vi "Front Panel Tyler.vi"() -> ()   [LabVIEW 2017, in "LD Reading.lvclass"]
uses:
  LD Reading.lvclass
  Reference Channel Intensities.ctl
  Sample Channel Intensities.ctl
  Realtime Output.ctl
  Average Data.ctl
  LD Reading.lvclass/LD Reading.ctl
  <vilib>/Utility/file.llb/Write Delimited Spreadsheet (string).vi
panel:
  out "Sample Averages":T1
  out "Reference Averages":T1
  in  "Export Data":bool
  out "Data Collection Progress":u8(slide) scale=0.0..100.0
  out "Current Phase":string
  in  "Data graphs":enum32{"Data", "Miscellaneous Data"}(tab)
  out "Diode/PMT":cluster{dbl[], dbl[]}(graph)
  out "RMS Voltage (mV)":cluster{dbl[], dbl[]}(graph)
  out "Photodiode Voltage  (V)":cluster{dbl[], dbl[]}(graph)
  out "PMT Voltage (V)":cluster{dbl[], dbl[]}(graph)
  in  "Data Collection Mode":enum32{"Reference", "Sample"}(radio)
  in  "Selected Sample Channel":enum32{"Channel 1", "Channel 2", "Channel 3"}(radio)
  in  "Selected Reference Channel":enum32{"Channel 1", "Channel 2", "Channel 3"}(radio)
  out "Realtime Output":T2
  out "Sample Analysis":T3
  out "Reference Analysis":T4
  in  "Correction Factor":dbl
  out "Finished":bool
  in  "Output Filename (stem)":path
  in  "Stop Data Collection":bool
  in  "Save Measurements?":bool
  out "Running":bool
  in  "Number of Data Points":dbl
  in  "Data Interval (s)":dbl
  in  "Collect Data":bool
  in  "stop":bool
  # "Data Collection Parameters"
  # "Experiment Control"
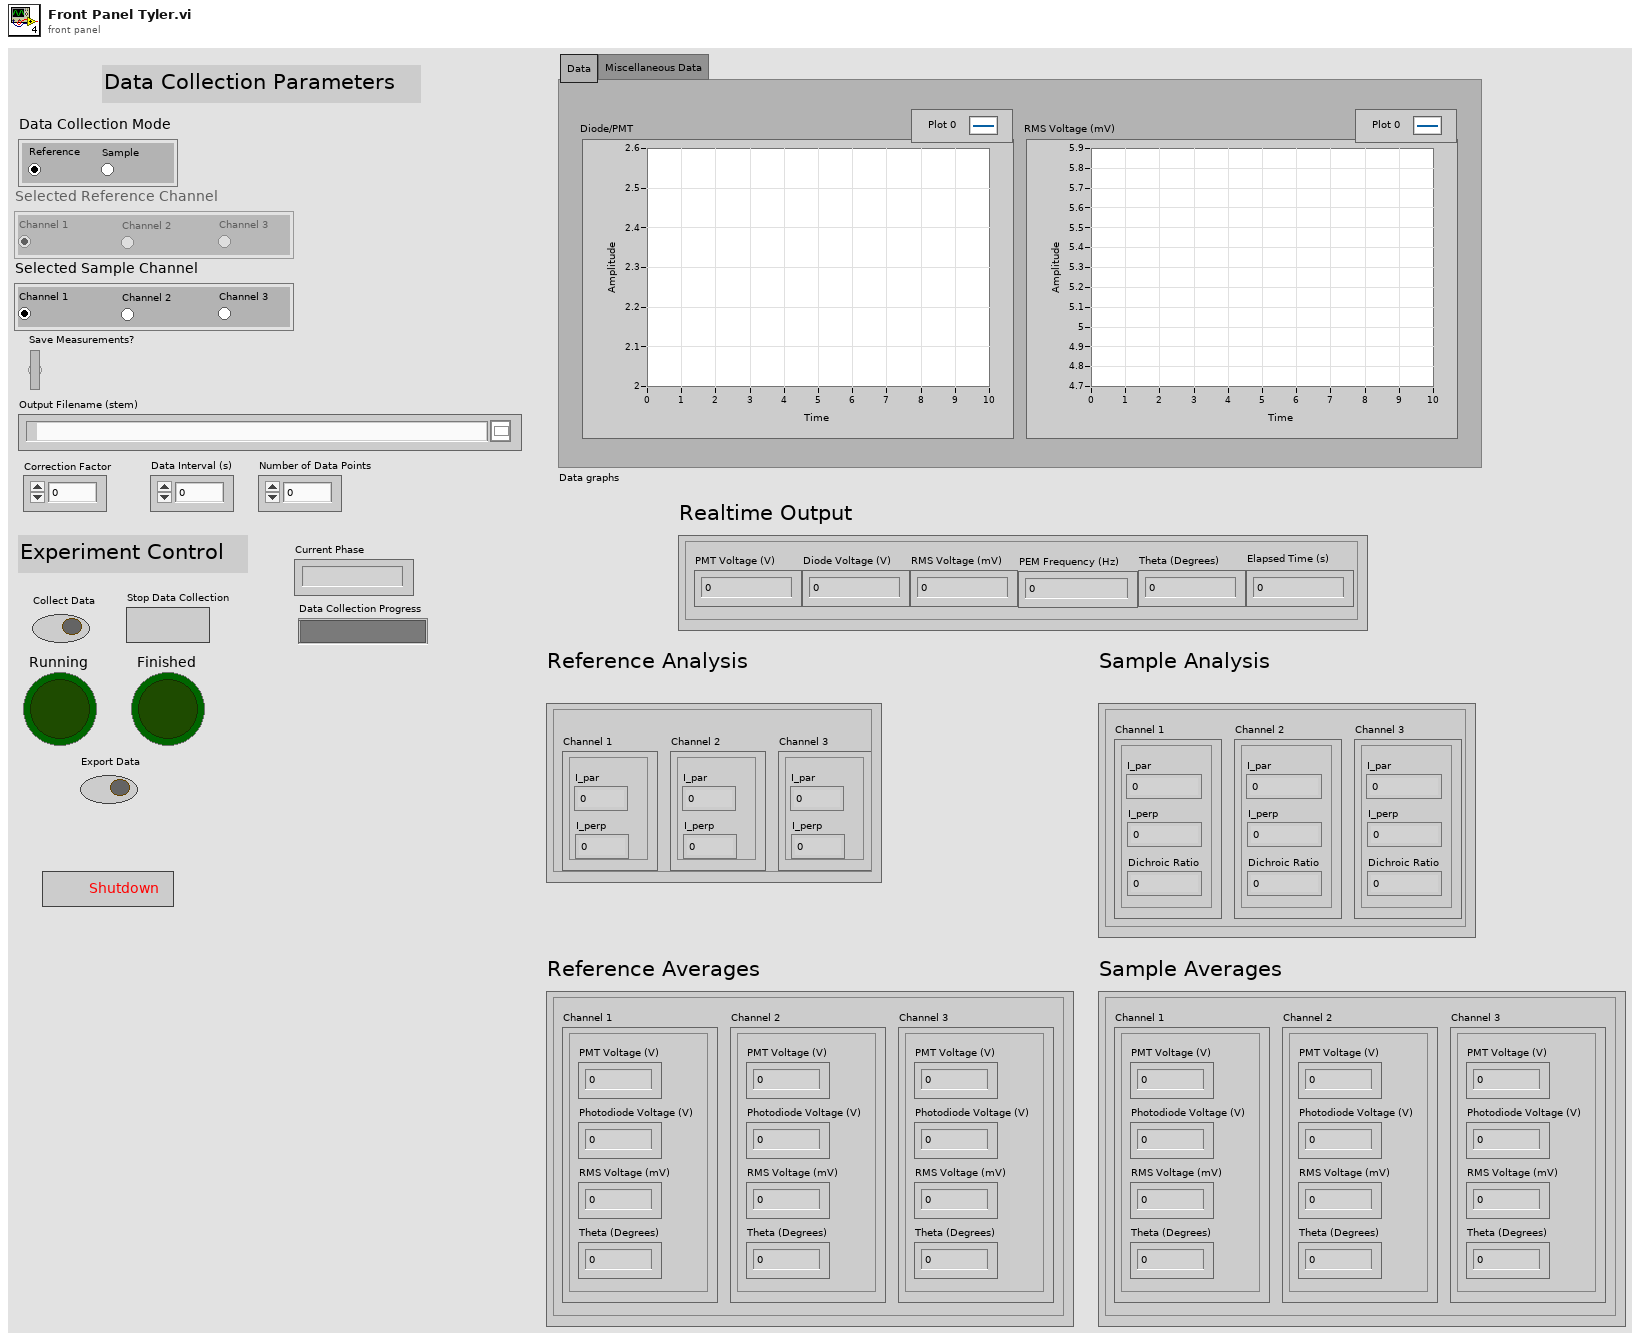
[diagram p1: front panel]
types:
  T1 = typedef "Average Data.ctl" = cluster{"Channel 1":cluster{"PMT Voltage (V)":dbl, "Photodiode Voltage (V)":dbl, "RMS Voltage (mV)":dbl, "Theta (Degrees)":dbl}, "Channel 2":cluster{"PMT Voltage (V)":dbl, "Photodiode Voltage (V)":dbl, "RMS Voltage (mV)":dbl, "Theta (Degrees)":dbl}, "Channel 3":cluster{"PMT Voltage (V)":dbl, "Photodiode Voltage (V)":dbl, "RMS Voltage (mV)":dbl, "Theta (Degrees)":dbl}}
  T2 = typedef "Realtime Output.ctl" = cluster{"Elapsed Time (s)":dbl, "PMT Voltage (V)":dbl, "Diode Voltage (V)":dbl, "RMS Voltage (mV)":dbl, "Theta (Degrees)":dbl, "PEM Frequency (Hz)":dbl}
  T3 = typedef "Sample Channel Intensities.ctl" = cluster{"Channel 1":cluster{"I_par":dbl, "I_perp":dbl, "Dichroic Ratio":dbl}, "Channel 2":cluster{"I_par":dbl, "I_perp":dbl, "Dichroic Ratio":dbl}, "Channel 3":cluster{"I_par":dbl, "I_perp":dbl, "Dichroic Ratio":dbl}}
  T4 = typedef "Reference Channel Intensities.ctl" = cluster{"Channel 1":cluster{"I_par":dbl, "I_perp":dbl}, "Channel 2":cluster{"I_par":dbl, "I_perp":dbl}, "Channel 3":cluster{"I_par":dbl, "I_perp":dbl}}
  T5 = enum8{"Enabled", "Disabled", "Disabled and Grayed Out"}
  T6 = cluster{dbl[], dbl[], dbl[], dbl[], dbl[], dbl[], dbl[]}
  T7 = cluster{"RMS Voltage Array":dbl[], "Photodiode Voltage Array":dbl[], "PMT Voltage Array":dbl[], "Diode/PMT Ratio Array":dbl[], "Time Array":dbl[], "PEM Frequency Array":dbl[], "Theta Array":dbl[]}
  T8 = cluster{"PMT Voltage (V)":dbl, "Photodiode Voltage (V)":dbl, "RMS Voltage (mV)":dbl, "Theta (Degrees)":dbl}
  T9 = cluster{"I_par":dbl, "I_perp":dbl, "Dichroic Ratio":dbl}
  T10 = typedef "NI_Matrix.lvlib/RealMatrix.ctl" = dbl[][]
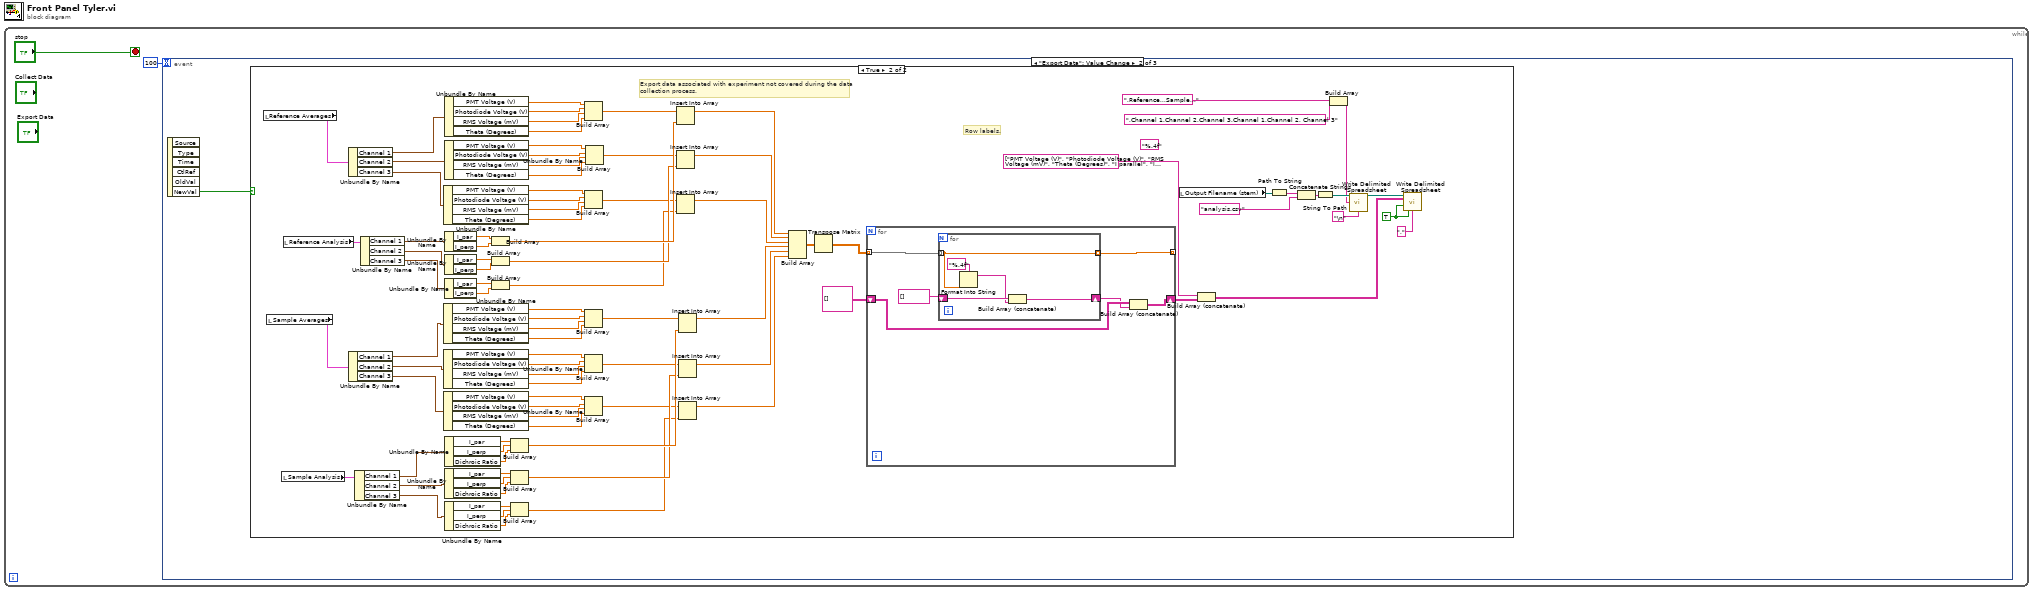
[diagram p0: block diagram]
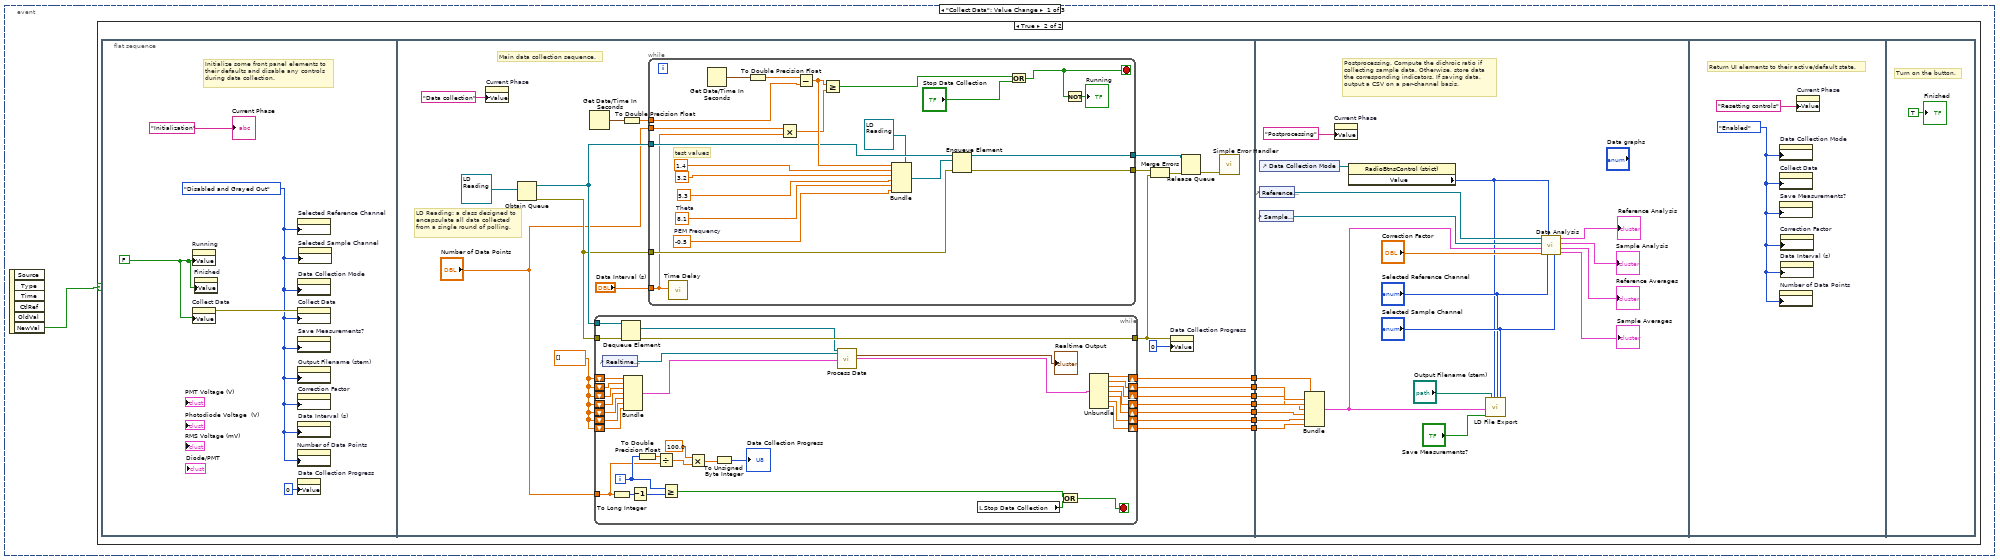
[diagram p2: hidden frame]
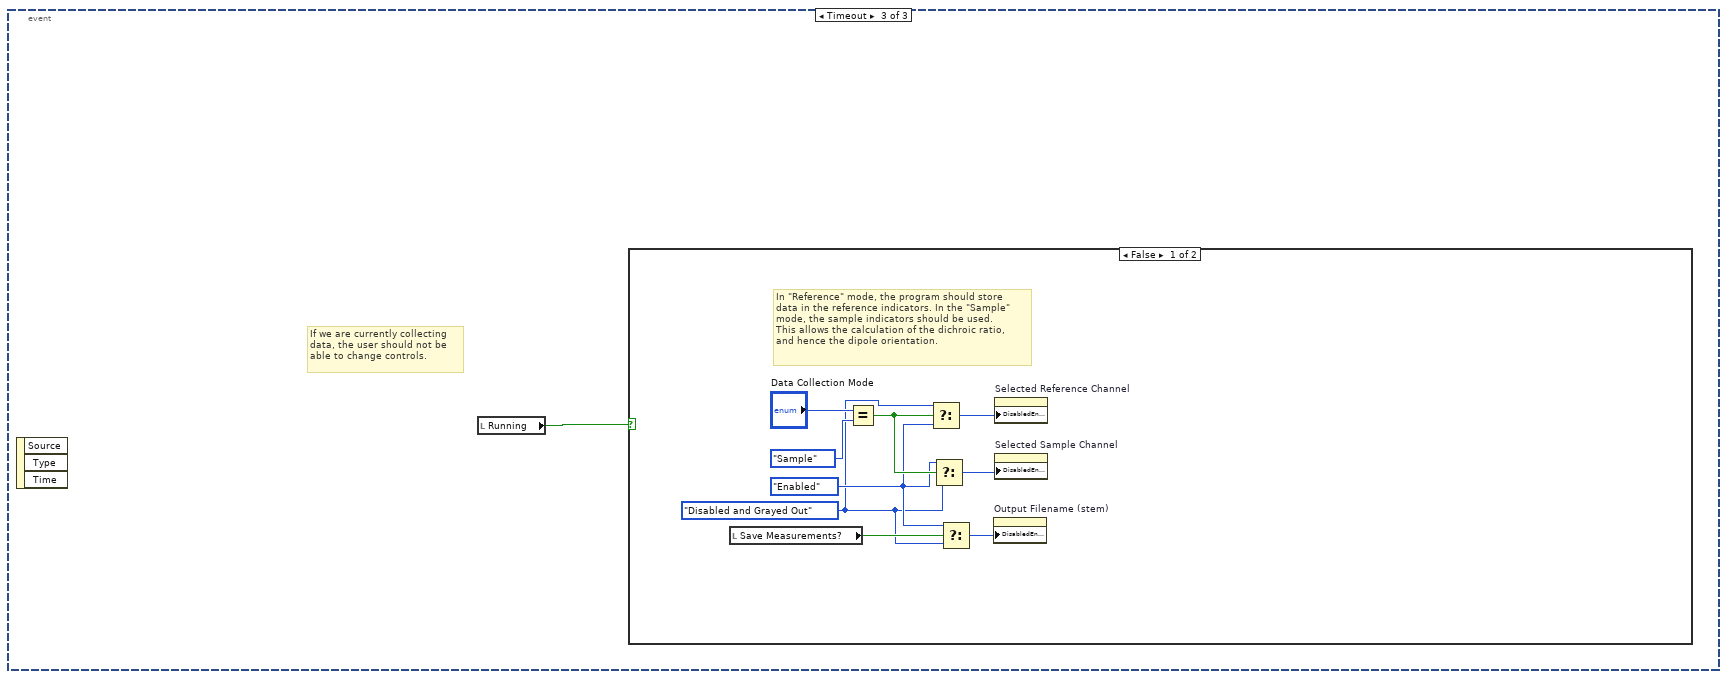
[diagram p5: hidden frame]
diagram:
  n1 = while {
    stop <- "stop" stop-if-true
    n2 = event shown="[1] \"Export Data\": Value Change" {
      selector: _ -> [_ _ _]
      dyn-events: _ -> [_ _ _]
      timeout: 100 -> [_ _ _]
      event "Collect Data": Value Change {
        n3 = event-data() -> ("NewVal"=w3:bool)  [unwired: 1 in, 5 out]
        n4 = case shown="True" w3 {
          frame False {
          }
          frame True {
            n5 = flat-sequence {
              tunnel: [w25] -> w10
              tunnel: [w24] -> w9
              tunnel: [w23] -> w8
              tunnel: [w26] -> w7
              tunnel: [w22] -> w6
              tunnel: [w21] -> w5
              tunnel: [w16] -> w4
              tunnel: w10 -> [w111]
              tunnel: w9 -> [w110]
              tunnel: w8 -> [w109]
              tunnel: w7 -> [w112]
              tunnel: w6 -> [w108]
              tunnel: w5 -> [w107]
              tunnel: w4 -> [w106]
              frame #0 {
                w13 = T5."Disabled and Grayed Out" ("Disabled")
                w15 = FALSE
                # "Initialize some front panel elements to \ntheir defaults and disable any controls \nduring data collection."
                n6 = property on="Running" class="Bool (strict)"("Value"=w15) -> ()  [unwired: 2 in, 2 out]
                n7 = property on="Collect Data" class="Bool (strict)"("Value"=w15) -> (error out=w14:errorcluster)  [unwired: 2 in, 1 out]
                n8 = property on="Finished" class="Bool (strict)"("Value"=w15) -> ()  [unwired: 2 in, 2 out]
                n9 = property on="Number of Data Points" class="DigNum (strict)"("DisabledEnum"=w13) -> ()  [unwired: 2 in, 2 out]
                n10 = property on="Selected Reference Channel" class="RadioBtnsControl (strict)"("DisabledEnum"=w13) -> ()  [unwired: 2 in, 2 out]
                n11 = property on="Data Collection Mode" class="RadioBtnsControl (strict)"("DisabledEnum"=w13) -> ()  [unwired: 2 in, 2 out]
                n12 = property on="Collect Data" class="Bool (strict)"(error in=w14, "DisabledEnum"=w13) -> ()  [unwired: 1 in, 2 out]
                n13 = property on="Save Measurements?" class="Bool (strict)"("DisabledEnum"=w13) -> ()  [unwired: 2 in, 2 out]
                n14 = property on="Output Filename (stem)" class="Path"("DisabledEnum"=w13) -> ()  [unwired: 2 in, 2 out]
                n15 = property on="Correction Factor" class="DigNum (strict)"("DisabledEnum"=w13) -> ()  [unwired: 2 in, 2 out]
                n16 = property on="Data Interval (s)" class="DigNum (strict)"("DisabledEnum"=w13) -> ()  [unwired: 2 in, 2 out]
                n17 = property on="Data Collection Progress" class="Slide (strict)"("Value"=u8 0 ("Progress")) -> ()  [unwired: 2 in, 2 out]
                n18 = property on="Selected Sample Channel" class="RadioBtnsControl (strict)"("DisabledEnum"=w13) -> ()  [unwired: 2 in, 2 out]
                "Current Phase" <- "Initialization"
              }
              frame #1 {
                w17 = dbl[] []
                # "Main data collection sequence."
                # "LD Reading: a class designed to \nencapsulate all data collected \nfrom a single round of polling."
                n19 = property on="Current Phase" class="Str"("Value"="Data collection") -> ()  [unwired: 2 in, 2 out]
                n20 = Obtain Queue(element data type=refnum<class "LD Reading.lvclass"> refnum ("LD Reading.lvclass")) -> (queue out=w33:refnum<queue>, error out=w32:errorcluster)  [unwired: 4 in, 1 out]
                n21 = Get Date/Time In Seconds() -> (seconds since 1Jan1904=w36:timestamp)
                n22 = while {
                  tunnel: w33 -> [w71]
                  shift-right: [w49] -> w26
                  shift-left: w17 -> [w56]
                  shift-right: [w48] -> w25
                  shift-left: w17 -> [w55]
                  shift-right: [w47] -> w24
                  shift-left: w17 -> [w54]
                  shift-right: [w46] -> w23
                  shift-left: w17 -> [w53]
                  shift-right: [w45] -> w22
                  shift-left: w17 -> [w52]
                  shift-right: [w44] -> w21
                  shift-left: w17 -> [w51]
                  shift-right: [w43] -> w16
                  shift-left: w17 -> [w50]
                  tunnel: w32 -> [w68]
                  tunnel: [w67] -> w19
                  tunnel: "Number of Data Points" -> [w57]
                  i -> [w62]
                  stop <- w70 stop-if-true
                  n23 = control-ref of="Realtime Output"() -> (w41:refnum<vi>)
                  n24 = To Long Integer(number=w57) -> (32bit integer=w63:i32)
                  n25 = Dequeue Element(queue=w71, error in (no error)=w68) -> (element=w42:refnum<class "LD Reading.lvclass">, error out=w67:errorcluster)  [unwired: 1 in, 2 out]
                  n26 = Bundle(w56, w55, w54, w53, w52, w51, w50) -> (w40:T6)  [unwired: 1 in]
                  n27 = Decrement(x=w63) -> (x-1=w66:i32)
                  n28 = To Double Precision Float(number=w62) -> (double precision float=w61:dbl)
                  n29 = Divide(x=w61, y=w57) -> (x/y=w64:dbl)
                  n30 = Greater Or Equal?(x=w62, y=w66) -> (x >= y?=w65:bool)
                  n31 = Multiply(x=100.0, y=w64) -> (x*y=w59:dbl)
                  n32 = To Unsigned Byte Integer(number=w59) -> (unsigned 8bit integer=→"Data Collection Progress":u8)
                  n33 = call "Process Data.vi"("LD Reading in"=w42, "reference"=w41, "Input Cluster"=w40) -> ("Realtime Output"=→"Realtime Output":T2, "Output Cluster"=w38:T7)  [unwired: 23 in]
                  n34 = local read "Stop Data Collection"() -> (w69:bool)
                  n35 = Or(x=w65, y=w69) -> (x .or. y?=w70:bool)
                  n36 = Unbundle(w38) -> ("RMS Voltage Array"=w49:dbl[], "Photodiode Voltage Array"=w48:dbl[], "PMT Voltage Array"=w47:dbl[], "Diode/PMT Ratio Array"=w46:dbl[], "Time Array"=w45:dbl[], "PEM Frequency Array"=w44:dbl[], "Theta Array"=w43:dbl[])
                }
                n37 = To Double Precision Float(number=w36) -> (double precision float=w35:dbl)
                n38 = while {
                  tunnel: "Data Interval (s)" -> [w74]
                  tunnel: w35 -> [w75]
                  tunnel: w33 -> [w84]
                  tunnel: [w81] -> w28
                  tunnel: w32 -> [w77]
                  tunnel: [w76] -> w31
                  tunnel: "Number of Data Points" -> [w73]
                  stop <- w78 stop-if-true
                  w85 = -0.5  # PEM Frequency
                  w86 = 8.1  # Theta
                  # "test values"
                  n39 = call "Time Delay"("Delay Time (s)"=w74) -> ()  [unwired: 10 in, 1 out]
                  n40 = Get Date/Time In Seconds() -> (seconds since 1Jan1904=w93:timestamp)
                  n41 = To Double Precision Float(number=w93) -> (double precision float=w92:dbl)
                  n42 = Multiply(x=w73, y=w74) -> (x*y=w72:dbl)
                  n43 = Subtract(x=w92, y=w75) -> (x-y=w88:dbl)
                  n44 = Greater Or Equal?(x=w88, y=w72) -> (x >= y?=w79:bool)
                  n45 = Bundle(cluster=refnum<class "LD Reading.lvclass"> refnum ("LD Reading.lvclass"), w88, 1.4 ("PMT Voltage"), 3.2 ("Diode Voltage"), 5.3 ("V_RMS"), w86, w85) -> (w82:refnum<class "LD Reading.lvclass">)
                  n46 = Enqueue Element(queue=w84, element=w82, error in (no error)=w77) -> (queue out=w81:refnum<queue>, error out=w76:errorcluster)  [unwired: 1 in, 1 out]
                  n47 = Or(x=w79, y="Stop Data Collection") -> (x .or. y?=w78:bool)
                  n48 = Not(x=w78) -> (.not. x?=→"Running":bool)
                }
                n49 = Merge Errors(w31, w19) -> (w30:errorcluster)
                n50 = property on="Data Collection Progress" class="Slide (strict)"(error in=w19, "Value"=u8 0 ("Progress")) -> ()  [unwired: 1 in, 2 out]
                n51 = Release Queue(queue=w28, error in (no error)=w30) -> (error out=w29:errorcluster)  [unwired: 1 in, 2 out]
                n52 = call <vilib>:"Simple Error Handler.vi"("error in (no error)"=w29) -> ()  [unwired: 4 in, 5 out]
              }
              frame #2 {
                # "Postprocessing. Compute the dichroic ratio if \ncollecting sample data. Otherwise, store data \nthe corresponding indicators. If saving data, \noutput a CSV on a per-channel basis."
                n53 = control-ref of="Data Collection Mode"() -> (w98:refnum<vi>)
                n54 = control-ref of="Sample Analysis"() -> (w101:refnum<vi>)
                n55 = control-ref of="Reference Analysis"() -> (w100:refnum<vi>)
                n56 = Bundle(w112, w111, w110, w109, w108, w107, w106) -> (w102:T6)  [unwired: 1 in]
                n57 = property on="Current Phase" class="Str"("Value"="Postprocessing") -> ()  [unwired: 2 in, 2 out]
                n58 = property class="RadioBtnsControl (strict)"(reference=w98) -> ("Value"=w96:enum32{"Reference", "Sample"})  [unwired: 1 in, 2 out]
                n59 = call "LD File Export.vi"("Input Cluster"=w102, "Save Data?"="Save Measurements?", "Output Filename (stem)"="Output Filename (stem)", "Data Collection Mode"=w96, "Selected Reference Channel"="Selected Reference Channel", "Selected Sample Channel"="Selected Sample Channel") -> ()  [unwired: 14 in]
                n60 = call "Data Analysis.vi"("Selected Sample Channel in"="Selected Sample Channel", "Selected Reference Channel in"="Selected Reference Channel", "Data Collection Mode"=w96, "Correction Factor"="Correction Factor", "Cluster"=w102, "Sample Indicator"=w101, "Reference Indicator"=w100) -> ("Sample Averages"=→"Sample Averages":T1, "Reference Averages"=→"Reference Averages":T1, "Sample Analysis"=→"Sample Analysis":T3, "Reference Analysis"=→"Reference Analysis":T4)  [unwired: 1 in]
              }
              frame #3 {
                w117 = T5."Enabled" ("Disabled")
                # "Return UI elements to their active/default state."
                n61 = property on="Data Collection Mode" class="RadioBtnsControl (strict)"("DisabledEnum"=w117) -> ()  [unwired: 2 in, 2 out]
                n62 = property on="Collect Data" class="Bool (strict)"("DisabledEnum"=w117) -> ()  [unwired: 2 in, 2 out]
                n63 = property on="Save Measurements?" class="Bool (strict)"("DisabledEnum"=w117) -> ()  [unwired: 2 in, 2 out]
                n64 = property on="Number of Data Points" class="DigNum (strict)"("DisabledEnum"=w117) -> ()  [unwired: 2 in, 2 out]
                n65 = property on="Correction Factor" class="DigNum (strict)"("DisabledEnum"=w117) -> ()  [unwired: 2 in, 2 out]
                n66 = property on="Data Interval (s)" class="DigNum (strict)"("DisabledEnum"=w117) -> ()  [unwired: 2 in, 2 out]
                n67 = property on="Current Phase" class="Str"("Value"="Resetting controls") -> ()  [unwired: 2 in, 2 out]
              }
              frame #4 {
                # "Turn on the button."
                "Finished" <- TRUE ("Finished")
              }
            }
          }
        }
      }
      event "Export Data": Value Change {
        n68 = event-data() -> ("NewVal"=w119:bool)  [unwired: 1 in, 5 out]
        n69 = case shown="True" w119 {
          frame False {
          }
          frame True {
            w121 = TRUE ("append to file? (new file:F)")
            (unwired) "%.4f" ("format string")
            # "Row labels."
            # "Export data associated with experiment not covered during the data \ncollection process."
            n70 = local read "Reference Averages"() -> (w203:T1)
            n71 = local read "Sample Averages"() -> (w201:T1)
            n72 = local read "Sample Analysis"() -> (w199:T3)
            n73 = local read "Reference Analysis"() -> (w207:T4)
            n74 = Unbundle By Name(w203) -> ("Channel 1"=w202:T8, "Channel 2"=w188:T8, "Channel 3"=w184:T8)
            n75 = Unbundle By Name(w201) -> ("Channel 1"=w172:T8, "Channel 2"=w163:T8, "Channel 3"=w162:T8)
            n76 = Unbundle By Name(w199) -> ("Channel 1"=w200:T9, "Channel 2"=w155:T9, "Channel 3"=w151:T9)
            n77 = Unbundle By Name(w207) -> ("Channel 1"=w206:cluster{"I_par":dbl, "I_perp":dbl}, "Channel 2"=w205:cluster{"I_par":dbl, "I_perp":dbl}, "Channel 3"=w204:cluster{"I_par":dbl, "I_perp":dbl})
            n78 = Unbundle By Name(w184) -> ("PMT Voltage (V)"=w174:dbl, "Photodiode Voltage (V)"=w187:dbl, "RMS Voltage (mV)"=w186:dbl, "Theta (Degrees)"=w185:dbl)
            n79 = Unbundle By Name(w172) -> ("PMT Voltage (V)"=w173:dbl, "Photodiode Voltage (V)"=w175:dbl, "RMS Voltage (mV)"=w176:dbl, "Theta (Degrees)"=w177:dbl)
            n80 = Unbundle By Name(w163) -> ("PMT Voltage (V)"=w171:dbl, "Photodiode Voltage (V)"=w170:dbl, "RMS Voltage (mV)"=w169:dbl, "Theta (Degrees)"=w168:dbl)
            n81 = Unbundle By Name(w162) -> ("PMT Voltage (V)"=w164:dbl, "Photodiode Voltage (V)"=w165:dbl, "RMS Voltage (mV)"=w166:dbl, "Theta (Degrees)"=w167:dbl)
            n82 = Unbundle By Name(w202) -> ("PMT Voltage (V)"=w196:dbl, "Photodiode Voltage (V)"=w195:dbl, "RMS Voltage (mV)"=w194:dbl, "Theta (Degrees)"=w193:dbl)
            n83 = Unbundle By Name(w188) -> ("PMT Voltage (V)"=w189:dbl, "Photodiode Voltage (V)"=w190:dbl, "RMS Voltage (mV)"=w191:dbl, "Theta (Degrees)"=w192:dbl)
            n84 = Unbundle By Name(w206) -> ("I_par"=w183:dbl, "I_perp"=w182:dbl)
            n85 = Unbundle By Name(w205) -> ("I_par"=w181:dbl, "I_perp"=w180:dbl)
            n86 = Unbundle By Name(w204) -> ("I_par"=w179:dbl, "I_perp"=w178:dbl)
            n87 = Unbundle By Name(w200) -> ("I_par"=w161:dbl, "I_perp"=w160:dbl, "Dichroic Ratio"=w159:dbl)
            n88 = Unbundle By Name(w155) -> ("I_par"=w156:dbl, "I_perp"=w157:dbl, "Dichroic Ratio"=w158:dbl)
            n89 = Unbundle By Name(w151) -> ("I_par"=w154:dbl, "I_perp"=w153:dbl, "Dichroic Ratio"=w152:dbl)
            n90 = Build Array(w183, w182) -> (w149:dbl[])
            n91 = Build Array(w181, w180) -> (w147:dbl[])
            n92 = Build Array(w179, w178) -> (w145:dbl[])
            n93 = Build Array(w161, w160, w159) -> (w143:dbl[])
            n94 = Build Array(w156, w157, w158) -> (w141:dbl[])
            n95 = Build Array(w154, w153, w152) -> (w139:dbl[])
            n96 = Build Array(w196, w195, w194, w193) -> (w150:dbl[])
            n97 = Build Array(w174, w187, w186, w185) -> (w146:dbl[])
            n98 = Build Array(w173, w175, w176, w177) -> (w144:dbl[])
            n99 = Build Array(w171, w170, w169, w168) -> (w142:dbl[])
            n100 = Build Array(w164, w165, w166, w167) -> (w140:dbl[])
            n101 = Build Array(w189, w190, w191, w192) -> (w148:dbl[])
            n102 = Insert Into Array(array=w150, new element=w149) -> (w138:dbl[])  [unwired: 1 in]
            n103 = Insert Into Array(array=w148, new element=w147) -> (w137:dbl[])  [unwired: 1 in]
            n104 = Insert Into Array(array=w146, new element=w145) -> (w136:dbl[])  [unwired: 1 in]
            n105 = Insert Into Array(array=w144, new element=w143) -> (w135:dbl[])  [unwired: 1 in]
            n106 = Insert Into Array(array=w142, new element=w141) -> (w134:dbl[])  [unwired: 1 in]
            n107 = Insert Into Array(array=w140, new element=w139) -> (w133:dbl[])  [unwired: 1 in]
            n108 = Build Array(w138, w137, w136, w135, w134, w133) -> (w126:T10)
            n109 = Transpose Matrix(1:w126) -> (0:w120:T10)
            n110 = for {
              tunnel: w120 -> [w216] mode=indexing
              tunnel: [w215] -> _ mode=indexing
              shift-right: [w211] -> w123
              shift-left: string[][] [] -> [w213]
              n111 = for {
                tunnel: w216 -> [w221] mode=indexing
                tunnel: [w221] -> w215 mode=indexing
                shift-right: [w217] -> w212
                shift-left: string[] [] -> [w219]
                n112 = Format Into String(format string="%.4f", w221) -> (resulting string=w218:string)  [unwired: 2 in, 1 out]
                n113 = Build Array (concatenate)(w219, w218) -> (w217:string[])
              }
              n114 = Build Array (concatenate)(w213, w212) -> (w211:string[][])
            }
            n115 = local read "Output Filename (stem)"() -> (w210:path)
            n116 = Build Array (concatenate)(string[] ["PMT Voltage (V)", "Photodiode Voltage (V)", "RMS Voltage (mV)", "Theta (Degrees)", "I parallel", "I perpendicular", "Dichroic Ratio"], w123) -> (w122:string[][])
            n117 = Path To String(path=w210) -> (string=w209:string)
            n118 = Concatenate Strings(w209, "analysis.csv") -> (w198:string)
            n119 = String To Path(string=w198) -> (path=w197:path)
            n120 = Build Array(",Reference,,,Sample,,,", ",Channel 1,Channel 2,Channel 3,Channel 1,Channel 2, Channel 3") -> (w128:string[])
            n121 = call-poly <vilib>:"Write Delimited Spreadsheet.vi"("file path (dialog if empty)"=w197, "1D data"=w128, "delimiter (\\t)"="\n" ("delimiter (\\t)")) -> ("new file path (Not A Path if cancelled)"=w132:path)  [unwired: 11 in, 1 out]
            n122 = call-poly <vilib>:"Write Delimited Spreadsheet.vi"("file path (dialog if empty)"=w132, "2D data"=w122, "append to file? (new file:F)"=w121, "transpose? (no:F)"=w121, "delimiter (\\t)"="," ("delimiter (\\t)")) -> ()  [unwired: 9 in, 2 out]
          }
        }
      }
      event Timeout {
        # "If we are currently collecting \ndata, the user should not be \nable to change controls."
        n123 = event-data() -> ()  [unwired: 1 in, 3 out]
        n124 = local read "Running"() -> (w222:bool)
        n125 = case shown="False" w222 {
          frame False {
            w223 = T5."Disabled and Grayed Out" ("Disabled")
            w224 = T5."Enabled" ("Disabled")
            # "In \"Reference\" mode, the program should store \ndata in the reference indicators. In the \"Sample\" \nmode, the sample indicators should be used. \nThis allows the calculation of the dichroic ratio, \nand hence the dipole orientation."
            n126 = local read "Save Measurements?"() -> (w225:bool)
            n127 = Equal?(x="Data Collection Mode", y=enum32{"Reference", "Sample"}."Sample") -> (x = y?=w230:bool)
            n128 = Select(t=w223, s=w230, f=w224) -> (s? t:f=w228:T5)
            n129 = Select(t=w224, s=w230, f=w223) -> (s? t:f=w227:T5)
            n130 = Select(t=w224, s=w225, f=w223) -> (s? t:f=w226:T5)
            n131 = property on="Output Filename (stem)" class="Path"("DisabledEnum"=w226) -> ()  [unwired: 2 in, 2 out]
            n132 = property on="Selected Reference Channel" class="RadioBtnsControl (strict)"("DisabledEnum"=w228) -> ()  [unwired: 2 in, 2 out]
            n133 = property on="Selected Sample Channel" class="RadioBtnsControl (strict)"("DisabledEnum"=w227) -> ()  [unwired: 2 in, 2 out]
          }
          frame True {
          }
        }
      }
    }
  }
